vi "Initiate.vi"(8 "error in (no error)":errorcluster, 9 "Include No-operation-pending Flag (True)":bool=TRUE, 10 "Initiation Option (0: Immediate)":i32(ring) items=["Immediate", "Continuous"], 11 "VISA resource name":refnum<visa-resource-name>) -> (0 "error out":errorcluster, 3 "VISA resource name out":refnum<visa-resource-name>)   [LabVIEW 2019, in "Keithley 6517.lvlib"]
doc: "Initiates the Model 6517B, and controls the no-operation-pending flag in the internal process of determining whether all pending operations of an initiate command are completed.\nAfter all programmed operations are completed, the instrument leaves the trigger layers and returns to the idle state if continuous initiation is disabled.\nContinuous initiation can be disabled by <b>Preset.vi</b>."
uses:
  Keithley 6517.lvlib
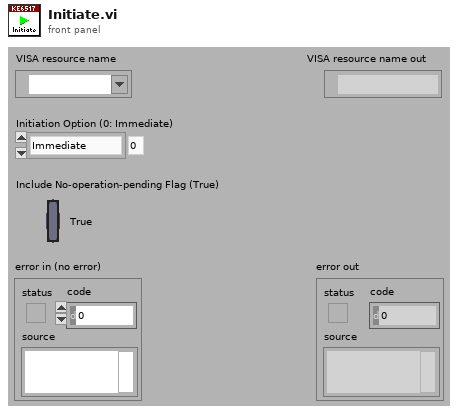
[diagram p1: front panel]
types:
  T1 = typedef "Keithley 6517.lvlib/Extended User Data.ctl" = cluster{"Instrument Model":i32}
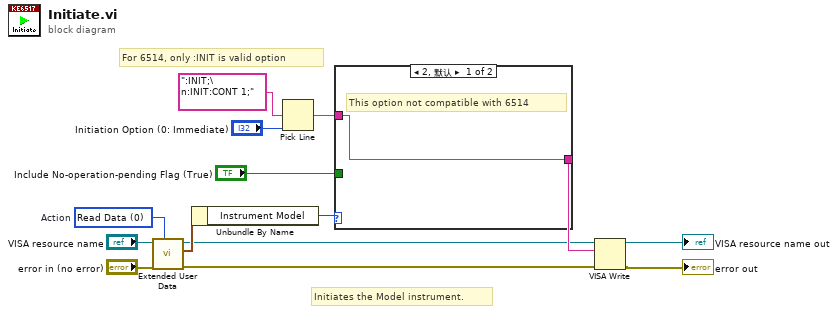
[diagram p0: block diagram]
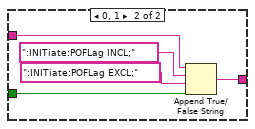
[diagram p2: hidden frame]
diagram:
  w10 = u16 0 items=["Read Data", "Write Data", "Clear Data", "Clear ALL Data"]  # Action
  # "For 6514, only :INIT is valid option"
  # "Initiates the Model instrument."
  n1 = call "Extended User Data.vi"("Action (0: Read Data)"=w10, "error in (no error)"="error in (no error)", "VISA resource name"="VISA resource name") -> ("error out"=w4:errorcluster, "User Data Out"=w6:T1, "VISA resource name out"=w5:refnum<visa-resource-name>)  [unwired: 6 in]
  n2 = Unbundle By Name(w6) -> ("Instrument Model"=w3:i32)
  n3 = Pick Line(multi-line string=":INIT;\n:INIT:CONT 1;", line index="Initiation Option (0: Immediate)") -> (output string=w7:string)  [unwired: 1 in]
  n4 = case shown="2, 默认" w3 {
    tunnel: "Include No-operation-pending Flag (True)" -> [_ w20]
    tunnel: [w15 w17] -> w13
    tunnel: w7 -> [w15 w16]
    frame 2, Default {
      # "This option not compatible with 6514"
    }
    frame 0, 1 {
      n5 = Append True/False String(1:w20, 2:":INITiate:POFLag EXCL;", 3:":INITiate:POFLag INCL;", 4:w16) -> (0:w17:string)
    }
  }
  n6 = VISA Write(VISA resource name=w5, write buffer=w13, error in (no error)=w4) -> (VISA resource name out=→"VISA resource name out":refnum<visa-resource-name>, error out=→"error out":errorcluster)  [unwired: 1 out]
